vi "Equi-Ripple BandPass (DBL).vi"(0 "X":dbl[](array[numeric]), 1 "lower pass freq":dbl=0.25000000000000006 format="%0.2f", 3 "# of taps":i32=32, 4 "lower stop freq":dbl=0.2 format="%0.2f", 5 "higher pass freq":dbl=0.3500000000000001 format="%0.2f", 8 "higher stop freq":dbl=0.4000000000000001 format="%0.2f", 9 "sampling freq: fs":dbl=1.0 format="%0.2f") -> (6 "Filtered X":dbl[](array[numeric]), 7 "error":i32)   [LabVIEW 2010, in "NI_AALBase.lvlib"]
doc: "Generates a bandpass FIR filter with equi-ripple characteristics using the Parks-McClellan algorithm and the <B>higher pass freq</B>, <B>lower pass freq</B>, <B># of taps</B>, <B>lower stop freq</B>, <B>higher stop freq</B>, and <B>sampling freq: fs</B>. The Equi-Ripple BandPass VI then applies a linear-phase, bandpass filter to the input sequence <B>X</B> using the Convolution VI to obtain <B>Filtered X</B>. Wire data to the <B>X</B> input to determine the polymorphic instance to use or manually select the instance."
uses:
  NI_AALBase.lvlib
  1D Convolution (DBL).vi
  NI_AALPro.lvlib
panel:
  # "Equi-Ripple\n Bandpass FIR Filter"
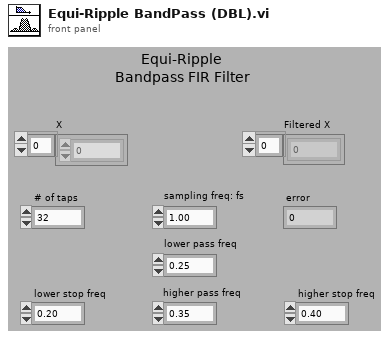
[diagram p1: front panel]
types:
  T1 = cluster{"Amplitude":dbl, "DC":dbl, "lower stop freq":dbl, "Weight":dbl}
  T2 = cluster{"Amplitude":dbl, "lower pass freq":dbl, "higher pass freq":dbl, "Weight":dbl}
  T3 = cluster{"Amplitude":dbl, "higher stop freq":dbl, dbl, "Weight":dbl}
  T4 = cluster{"Amplitude":dbl, "higher stop freq":dbl, "higher pass freq":dbl, "Weight":dbl}[]
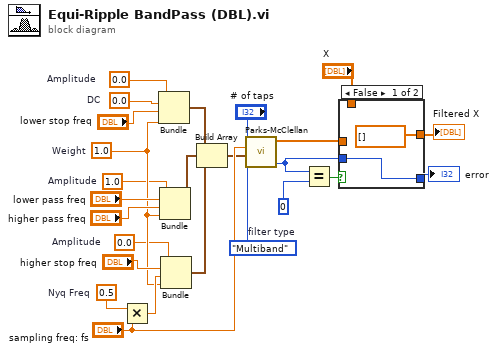
[diagram p0: block diagram]
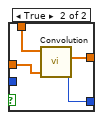
[diagram p2: hidden frame]
diagram:
  w11 = enum32{"Multiband", "Differentiator", "Hilbert"}."Multiband"  # filter type
  w2 = 0.0  # Amplitude
  w1 = 0.5  # Nyq Freq
  w3 = 1.0  # Amplitude
  w4 = 1.0  # Weight
  w5 = 0.0  # DC
  w6 = 0.0  # Amplitude
  n1 = Multiply(x=w1, y="sampling freq: fs") -> (x*y=w15:dbl)
  n2 = Bundle("Amplitude"=w6, "DC"=w5, "lower stop freq"="lower stop freq", "Weight"=w4) -> (w23:T1)  [unwired: 1 in]
  n3 = Bundle("Amplitude"=w3, "lower pass freq"="lower pass freq", "higher pass freq"="higher pass freq", "Weight"=w4) -> (w22:T2)  [unwired: 1 in]
  n4 = Bundle("Amplitude"=w2, "higher stop freq"="higher stop freq", w15, "Weight"=w4) -> (w14:T3)  [unwired: 1 in]
  n5 = Build Array(w23, w22, w14) -> (w12:T4)
  n6 = call "Parks-McClellan.vi"("filter type"=w11, "Band Parameters"=w12, "sampling freq: fs"="sampling freq: fs", "# of taps"="# of taps") -> ("error"=w8:i32, "h"=w10:dbl[])  [unwired: 1 out]
  n7 = Equal?(x=w8, y=0) -> (x = y?=w9:bool)
  n8 = case shown="False" w9 {
    tunnel: w8 -> [w27 _]
    tunnel: [w27 w28] -> w21
    tunnel: [dbl[] [] ("empty array") w29] -> w20
    tunnel: "X" -> [_ w31]
    tunnel: w10 -> [_ w30]
    frame False {
    }
    frame True {
      n9 = call-poly "Convolution.vi"("Y"=w30, "X"=w31) -> ("error"=w28:i32, "X * Y"=w29:dbl[])  [unwired: 8 in]
    }
  }
  "Filtered X" <- w20
  "error" <- w21
